vi "FisherPaykel Add CS CR.vi"(8 "Error In":errorcluster, 11 "Command Input":string) -> (0 "Error Out":errorcluster, 3 "Command w/ [CS] [CR]":string)   [LabVIEW 2016]
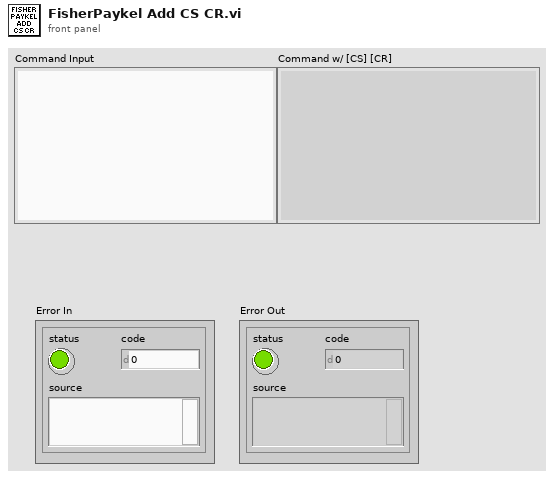
[diagram p1: front panel]
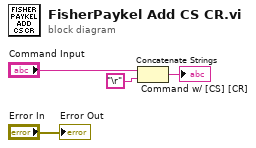
[diagram p0: block diagram]
diagram:
  n1 = Concatenate Strings("Command Input", "\r") -> (→"Command w/ [CS] [CR]":string)
  "Error Out" <- "Error In"
